vi "CreateTestPlot(SubVI).vi"(8 "Error In":errorcluster) -> (0 "Error Out":errorcluster, 3 "Result String":string)   [LabVIEW 2018]
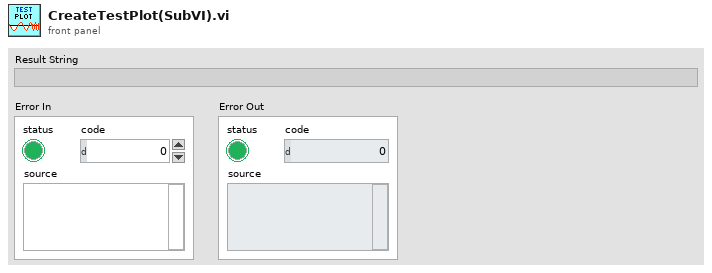
[diagram p1: front panel]
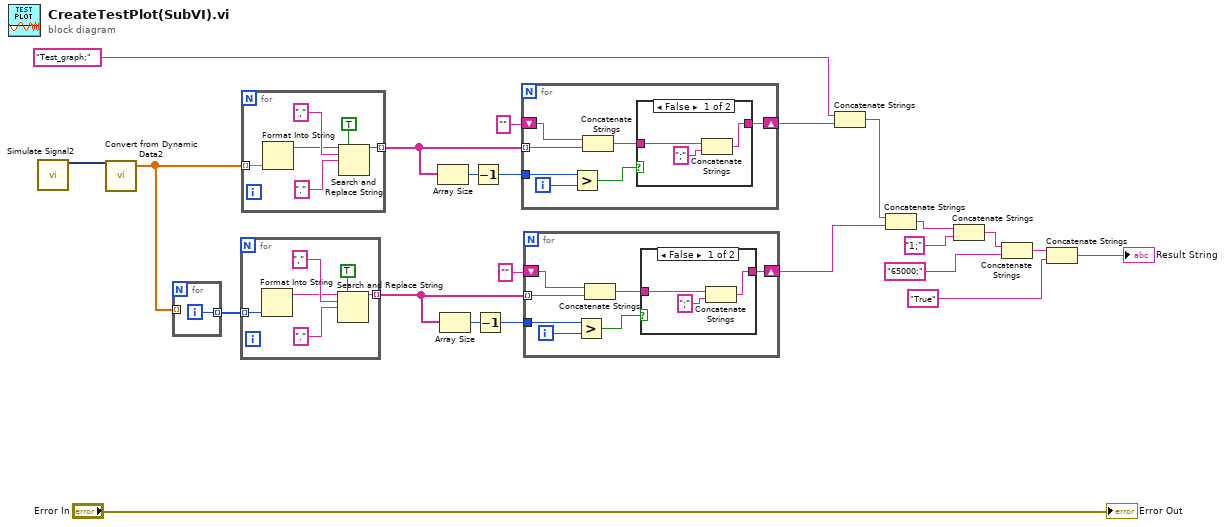
[diagram p0: block diagram]
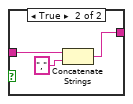
[diagram p2: hidden frame]
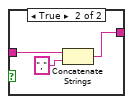
[diagram p3: hidden frame]
diagram:
  n1 = call "Simulate Signal2"() -> ("Sine with Uniform Noise"=w23:dynamicdata)  [unwired: 14 in, 1 out]
  n2 = call "Convert from Dynamic Data2"("Dynamic Data Type"=w23) -> ("Array"=w1:dbl[])  [unwired: 3 in]
  n3 = for {
    tunnel: [w24] -> w22 mode=indexing
    tunnel: w1 -> [_] mode=indexing
    i -> [w24]
  }
  n4 = for {
    tunnel: w22 -> [w30] mode=indexing
    tunnel: [w25] -> w14 mode=indexing
    n5 = Format Into String(w30) -> (resulting string=w26:string)  [unwired: 3 in, 1 out]
    n6 = Search and Replace String(replace all?=TRUE ("replace all? (F)"), input string=w26, search string=",", replace string="." ("replace string (\"\")")) -> (result string=w25:string)  [unwired: 4 in, 3 out]
  }
  n7 = for {
    tunnel: w1 -> [w36] mode=indexing
    tunnel: [w31] -> w18 mode=indexing
    n8 = Format Into String(w36) -> (resulting string=w32:string)  [unwired: 3 in, 1 out]
    n9 = Search and Replace String(replace all?=TRUE ("replace all? (F)"), input string=w32, search string=",", replace string="." ("replace string (\"\")")) -> (result string=w31:string)  [unwired: 4 in, 3 out]
  }
  n10 = Array Size(array=w18) -> (size(s)=w20:i32)
  n11 = Array Size(array=w14) -> (size(s)=w16:i32)
  n12 = Decrement(x=w20) -> (x-1=w19:i32)
  n13 = Decrement(x=w16) -> (x-1=w15:i32)
  n14 = for {
    tunnel: w18 -> [w40] mode=indexing
    shift-right: [w41] -> w13
    shift-left: "" -> [w43]
    tunnel: w19 -> [w37]
    i -> [w38]
    n15 = Greater?(x=w37, y=w38) -> (0:w39:bool)
    n16 = Concatenate Strings(w43, w40) -> (w42:string)
    n17 = case shown="False" w39 {
      tunnel: w42 -> [w45 w48]
      tunnel: [w44 w47] -> w41
      frame False {
        n18 = Concatenate Strings(w45, ";" ("string")) -> (w44:string)
      }
      frame True {
        n19 = Concatenate Strings(w48, "," ("string")) -> (w47:string)
      }
    }
  }
  n20 = for {
    tunnel: w14 -> [w53] mode=indexing
    shift-right: [w54] -> w11
    shift-left: "" -> [w56]
    tunnel: w15 -> [w50]
    i -> [w51]
    n21 = Greater?(x=w50, y=w51) -> (0:w52:bool)
    n22 = Concatenate Strings(w56, w53) -> (w55:string)
    n23 = case shown="False" w52 {
      tunnel: w55 -> [w58 w61]
      tunnel: [w57 w60] -> w54
      frame False {
        n24 = Concatenate Strings(w58, ";" ("string")) -> (w57:string)
      }
      frame True {
        n25 = Concatenate Strings(w61, "," ("string")) -> (w60:string)
      }
    }
  }
  n26 = Concatenate Strings("Test_graph;" ("string"), w13) -> (w12:string)
  n27 = Concatenate Strings(w12, w11) -> (w10:string)
  n28 = Concatenate Strings(w10, "1;" ("string")) -> (w7:string)
  n29 = Concatenate Strings(w7, "65000;" ("string")) -> (w5:string)
  n30 = Concatenate Strings(w5, "True" ("string")) -> (→"Result String":string)
  "Error Out" <- "Error In"
